vi "Example Test 1.vi"() -> ()   [LabVIEW 2014]
uses:
  Arduino MPU6050.lvlib
panel:
  in  "Error In":errorcluster
  out "error out":errorcluster
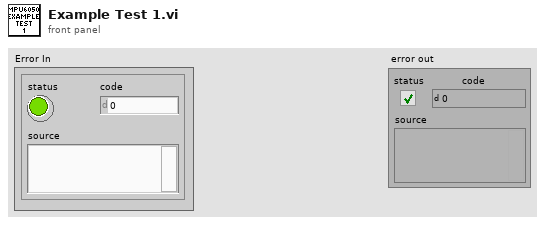
[diagram p1: front panel]
types:
  T1 = typedef "Arduino MPU6050.lvlib/Vector Datatype.ctl" = cluster{"XAxis":dbl, "YAxis":dbl, "ZAxis":dbl}
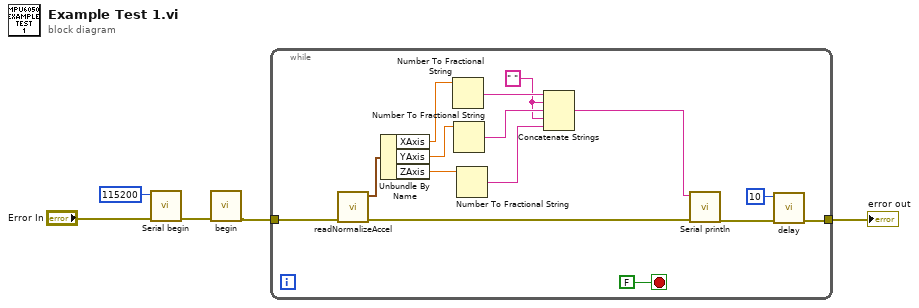
[diagram p0: block diagram]
diagram:
  n1 = call <vilib>:"Serial begin.vi"("Error In"="Error In", "speed (Bd)"=115200) -> ("Error Out"=w3:errorcluster)  [unwired: 9 in]
  n2 = call "begin.vi"("Error In"=w3) -> ("Error Out"=w4:errorcluster)  [unwired: 10 in]
  n3 = while {
    tunnel: w4 -> [w20]
    tunnel: [w14] -> w5
    stop <- FALSE stop-if-true
    w6 = " " ("F-format string")
    n4 = call "readNormalizeAccel.vi"("error in (no error)"=w20) -> ("error out"=w11:errorcluster, "Vector"=w19:T1)  [unwired: 9 in]
    n5 = Unbundle By Name(w19) -> ("XAxis"=w17:dbl, "YAxis"=w16:dbl, "ZAxis"=w15:dbl)
    n6 = Number To Fractional String(number=w17) -> (F-format string=w10:string)  [unwired: 3 in]
    n7 = Number To Fractional String(number=w16) -> (F-format string=w9:string)  [unwired: 3 in]
    n8 = Number To Fractional String(number=w15) -> (F-format string=w8:string)  [unwired: 3 in]
    n9 = Concatenate Strings(w10, w6, w9, w6, w8) -> (w7:string)
    n10 = call <vilib>:"Serial println.vi"("Error In"=w11, "string in"=w7) -> ("Error Out"=w13:errorcluster)  [unwired: 9 in]
    n11 = call <vilib>:"delay.vi"("Error In"=w13, "time (ms)"=10) -> ("Error Out"=w14:errorcluster)  [unwired: 9 in]
  }
  "error out" <- w5
